vi "Simulation - Windows plant only.vi"() -> ()   [LabVIEW 2025]
doc: "This example demonstrates a process simulation for a tank level. The process has added noise, valve deadband, lag, and deadtime. A level controller adjusts the inflow to a tank. An on/off valve serves as a drain that you can click on to operate. This s-valve represents a change in the process loading. You also can switch this VI from automatic control to manual control."
uses:
  <vilib>/addons/control/pid/pid.llb/PID Advanced (DBL).vi
  <vilib>/addons/control/pid/NI_PID_pid.lvlib
panel:
  in  "Physical Model":bool=TRUE
  in  "Tab Control":enum32{"Introduction", "Operation"}(tab)=enum."Operation"
  out "Flow sensor":bool
  in  "HV-101":bool
  out "tank level":dbl(slide) scale=0.0..100.0 scale format="%#.2g"
  out "Valve":bool
  in  "LCV-101":dbl(knob) scale=0.0..100.0
  in  "Auto":bool=TRUE
  out "Process Chart":T1(graph)={"initial PV"=18.934717983735947, "SP(%)"=34.59119496855346, "output"=100.0}
  in  "Setpoint":dbl(slide)=50.0 scale=0.0..100.0
  in  "PID parameters (LIC 101)":T2={"Kc"=10.0, "Ti (min)"=0.05, "Td (min)"=0.0} {"Td (min)" format="%#.6f"; "Ti (min)" format="%#.4f"; "Kc" format="%#.4f"}
  in  "Stop":bool
  # "Tank Level Control"
  # "Overview: This example demonstrates a process simulation for a tank level.  The process has added noise, valve deadband, lag, and deadtime.  A level controller adjusts the inflow to a tank.  An on/off valve serves as a drain that you can click on to operate.  This s-valve represents a change in the process loading.  You also can switch this VI from automatic control to manual control.\nInstructions:\n1. Run the VI.\n2. Verify the PID controller in closed-loop to track the setpoint.\n3. Change the setpoint to another value and verify the controller tracking the new setpoint.\n4. Apply a disturbance to the system by switching the valve HV 102 (click on the valve symbol). You will see the controller recovering fro the change.\n5. Change PID gains and see if you can improve its performance without going unstable.\n6. Switch to manual mode and see if you can control the level by changing the Valve LVC 101.\n7. Click Stop to stop the VI."
  # "ISA Symbology: The diagram uses the ISA Symbology used for control"
  # "Loop 101"
  # "Level Controller at the control room"
  # "Level Transmitter on the field"
  # "Level Control Valve on the field"
  # "Hand Control Valve on the field"
  # "HV"
  # "102"
  # "LCV"
  # "101"
  # "LIC"
  # "101"
  # "LT"
  # "101"
  # "Slow Leak"
  # "Click to operate"
  # "HV"
  # "102"
  # "LCV"
  # "101"
  # "LIC"
  # "101"
  # "LT"
  # "101"
  # "Manual"
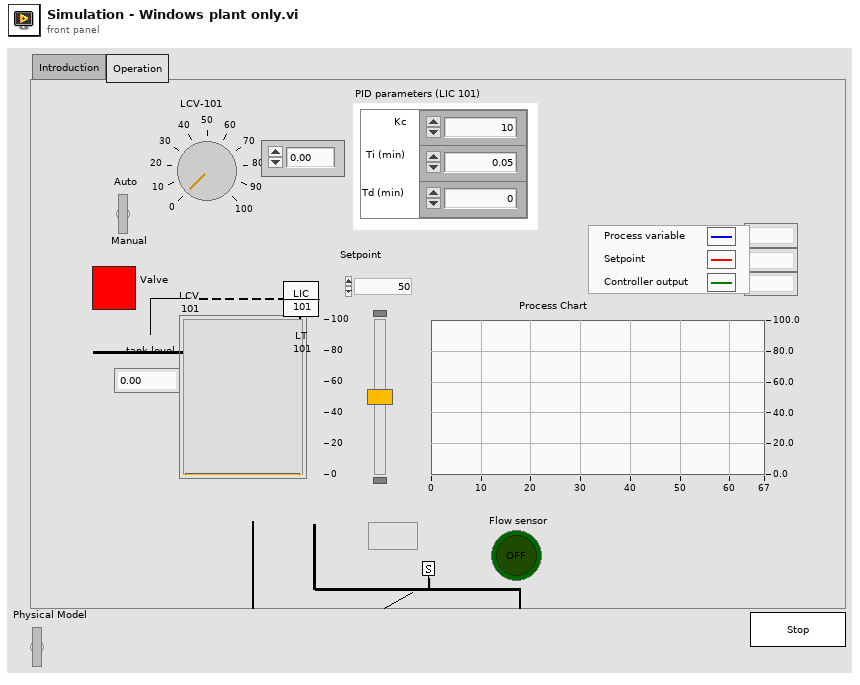
[diagram p1: front panel]
types:
  T1 = cluster{"initial PV":dbl, "SP(%)":dbl, "output":dbl}
  T2 = cluster{"Kc":dbl, "Ti (min)":dbl, "Td (min)":dbl}
  T3 = cluster{"static gain":dbl, "lag (s)":dbl, "deadtime (s)":dbl, "load":dbl, "deadband":dbl, "sensor noise":dbl, "initial PV":dbl, "plant noise":dbl}
  T4 = cluster{"Plant Output":dbl, "Setpoint":dbl, "output":dbl}
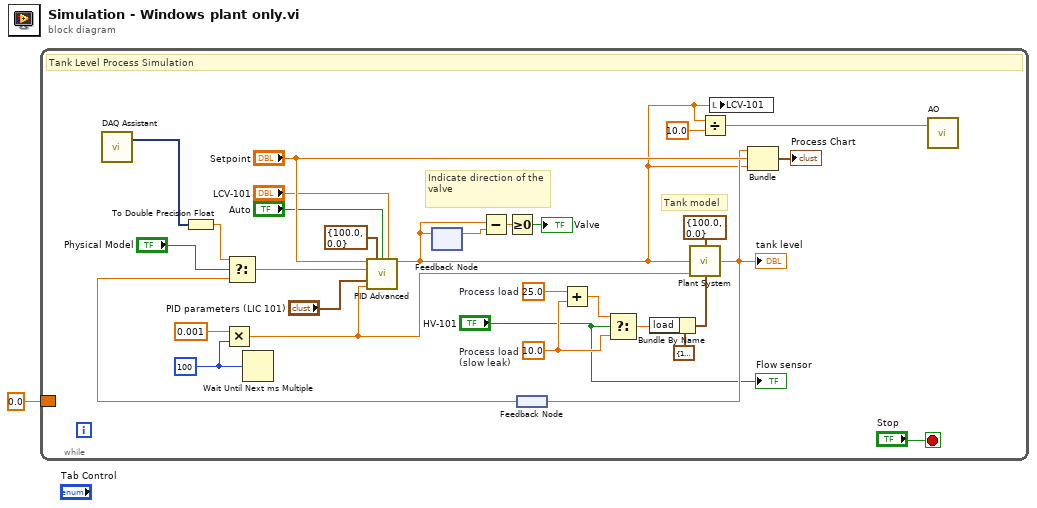
[diagram p0: block diagram]
diagram:
  n1 = while {
    border: 0.0 ("Plant Output") -> [_]
    stop <- "Stop" stop-if-true
    w19 = u32 100
    w12 = 25.0  # Process load
    w13 = 10.0  # Process load (slow leak)
    # "Tank model"
    # "Indicate direction of the valve"
    # "Tank Level Process Simulation"
    n2 = call "DAQ Assistant"() -> ("data"=w2:dynamicdata)  [unwired: 17 in, 2 out]
    n3 = To Double Precision Float(number=w2) -> (double precision float=w3:dbl)
    n4 = Multiply(x=0.001, y=w19) -> (x*y=w18:dbl)
    n5 = Wait Until Next ms Multiple(millisecond multiple=w19) -> ()  [unwired: 1 out]
    n6 = feedback #1() -> (w16:dbl)  [unwired: 1 in]
    n7 = feedback #2() -> (w5:dbl)
    n8 = Select(t=w3, s="Physical Model", f=w5) -> (s? t:f=w6:dbl)
    n9 = call-poly <vilib>:"PID Advanced.vi"("setpoint"="Setpoint", "output range"=cluster{"output high":dbl, "output low":dbl} {"output high"=100.0, "output low"=0.0}, "auto? (T)"="Auto", "manual control"="LCV-101", "process variable"=w6, "PID gains"="PID parameters (LIC 101)", "dt (s)"=w18) -> ("output"=w9:dbl)  [unwired: 7 in, 1 out]
    n10 = feedback-in #1(w9) -> ()
    n11 = Subtract(x=w9, y=w16) -> (x-y=w15:dbl)
    n12 = Greater Or Equal To 0?(x=w15) -> (x >= 0?=→"Valve":bool)
    n13 = Add(x=w12, y=w13) -> (x+y=w11:dbl)
    n14 = Select(t=w11, s="HV-101", f=w13) -> (s? t:f=w22:dbl)
    n15 = Bundle By Name(cluster=T3 {"static gain"=1.5, "lag (s)"=18.0, "deadtime (s)"=1.0, "load"=0.0, "deadband"=1.0, "sensor noise"=0.0, "initial PV"=0.0, "plant noise"=5.0} ("process parameters"), "load"=w22) -> (w21:T3)
    n16 = call "Plant System.vi"("output saturation range"=cluster{"output high":dbl, "output low":dbl} {"output high"=100.0, "output low"=0.0}, "Plant Input"=w9, "dt (s)"=w18, "process parameters"=w21) -> ("Plant Output"=w17:dbl)  [unwired: 11 in]
    "tank level" <- w17
    n17 = feedback-in #2(w17) -> ()
    n18 = Divide(x=w9, y=10.0) -> (x/y=w7:dbl)
    n19 = local write "LCV-101"(w9) -> ()
    n20 = Bundle("Plant Output"=w17, "Setpoint"="Setpoint", "output"=w9) -> (→"Process Chart":T4)  [unwired: 1 in]
    n21 = call "AO"("data"=w7) -> ()  [unwired: 17 in, 2 out]
    "Flow sensor" <- "HV-101"
  }
